vi "Get Next Step.vi"(8 "error in (no error)":errorcluster, 11 "Sequencer in":refnum<class "Sequencer.lvclass">) -> (0 "error out":errorcluster, 3 "Next Step":u32)   [LabVIEW 2024, in "Ramses Sequencer.lvlib" / "Sequencer.lvclass"]
uses:
  Sequencer.lvclass
  C:/Program Files (x86)/Enterative/Ramses Framework/Ramses Framework.lvlibp/Service/Service.lvclass
  Program Files (x86)/Enterative/Ramses Framework/Ramses Framework.lvlibp/Service/Service.lvclass
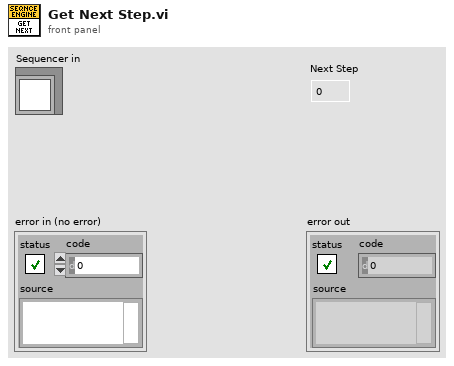
[diagram p1: front panel]
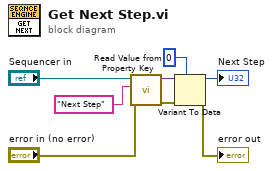
[diagram p0: block diagram]
diagram:
  n1 = call "Read Value from Property Key.vi"("error in (no error)"="error in (no error)", "Key"="Next Step", "Service in"="Sequencer in") -> ("error out"=w3:errorcluster, "Value"=w4:variant)  [unwired: 7 in]
  n2 = Variant To Data(error in=w3, type=u32 0, Variant=w4) -> (data=→"Next Step":u32, error out=→"error out":errorcluster)
